vi "SendStartUpInitStatus.vi"(8 "error in (no error)":errorcluster, 10 "EDP Startup Init Status":T1, 11 "Handle In":u32 format="%x") -> (0 "error out":errorcluster, 3 "Handle Out":u32 format="%x")   [LabVIEW 2020]
uses:
  <userlib>/Beckhoff-LabVIEW-Interface/_DependsOn/With TypeResolving/Write Sync Single TypeResolved.vi
panel:
  in  "WriteGrpSymbols 2":string[](array[string])=["192.168.0.20.1.1:851::GVL_LabviewDataShare.in_bAardvarkBoardError_labview", "192.168.0.20.1.1:851::GVL_LabviewDataShare.in_bAsic1CalibrationCompleted_labview", "192.168.0.20.1.1:851::GVL_LabviewDataShare.in_bAsic1CalibrationInProgress_labview", "192.168.0.20.1.1:851::GVL_LabviewDataShare.in_bAsic1CalibrationSuccess_labview", "192.168.0.20.1.1:851::GVL_LabviewDataShare.in_bAsic1FFTCompleted_labview", "192.168.0.20.1.1:851::GVL_LabviewDataShare.in_bAsic1FFTInProgress_labview", "192.168.0.20.1.1:851::GVL_LabviewDataShare.in_bAsic1FFTSuccess_labview", "192.168.0.20.1.1:851::GVL_LabviewDataShare.in_bAsic2CalibrationCompleted_labview", "192.168.0.20.1.1:851::GVL_LabviewDataShare.in_bAsic2CalibrationInProgress_labview", "192.168.0.20.1.1:851::GVL_LabviewDataShare.in_bAsic2CalibrationSuccess_labview", "192.168.0.20.1.1:851::GVL_LabviewDataShare.in_bAsic2FFTCompleted_labview", "192.168.0.20.1.1:851::GVL_LabviewDataShare.in_bAsic2FFTInProgress_labview", "192.168.0.20.1.1:851::GVL_LabviewDataShare.in_bAsic2FFTSuccess_labview", "192.168.0.20.1.1:851::GVL_LabviewDataShare.in_bCalResultsDBStoreSuccess_labview", "192.168.0.20.1.1:851::GVL_LabviewDataShare.in_bFFTResultsDBStoreSuccess_labview", "192.168.0.20.1.1:851::GVL_LabviewDataShare.in_bLabviewHandshakeBit", "192.168.0.20.1.1:851::GVL_LabviewDataShare.in_bLabviewResetComplete_labview", "192.168.0.20.1.1:851::GVL_LabviewDataShare.in_bLabviewResetSuccess_labview", "192.168.0.20.1.1:851::GVL_LabviewDataShare.in_bNIDaqError_labview", "192.168.0.20.1.1:851::GVL_LabviewDataShare.in_bPTC04BoardError_labview", "192.168.0.20.1.1:851::GVL_LabviewDataShare.in_bStartupInitializationCompleted_labview", "192.168.0.20.1.1:851::GVL_LabviewDataShare.in_bStartupInitializationSuccess_labview", "192.168.0.20.1.1:851::GVL_LabviewDataShare.in_strAsic1SerialNo_labview", "192.168.0.20.1.1:851::GVL_LabviewDataShare.in_strAsic2SerialNo_labview"]
  out "Write Status 2":bool
  out "Has Matched? 2":bool
  out "Write Status":bool
  out "Has Matched?":bool
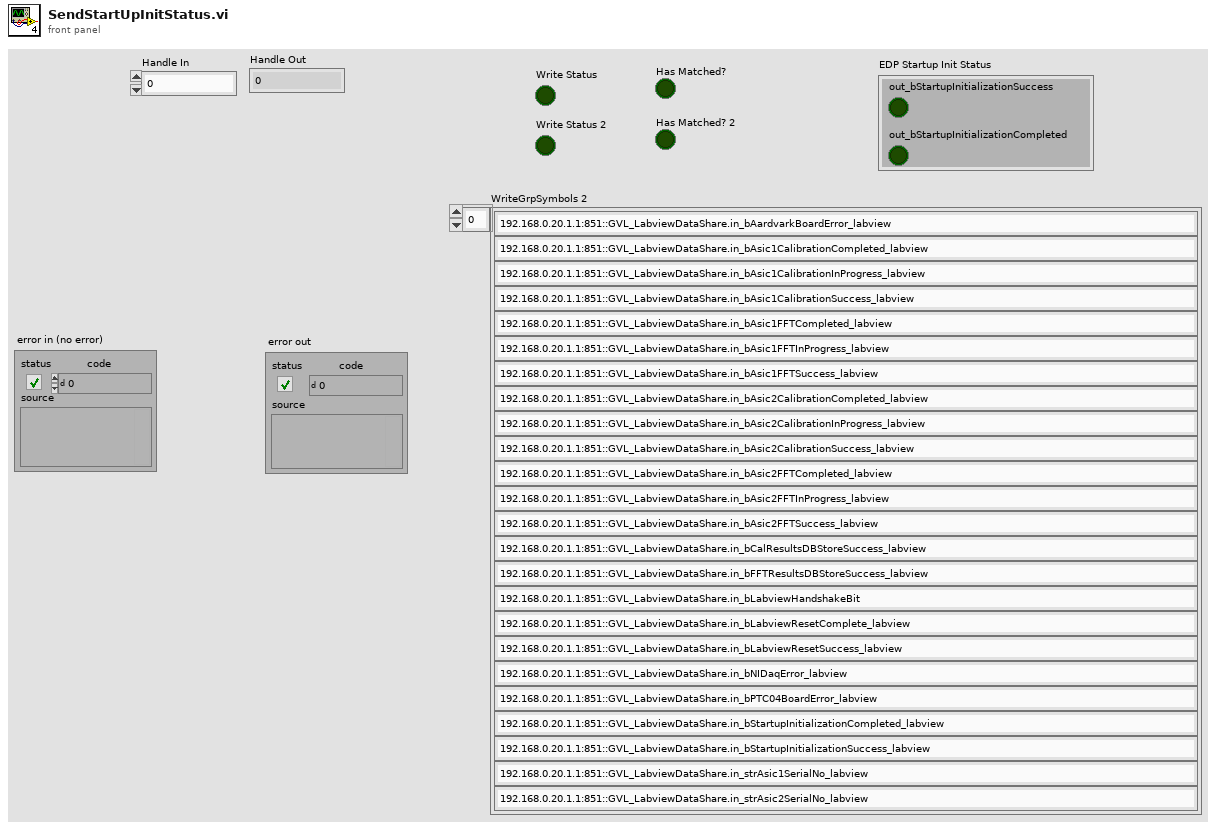
[diagram p1: front panel]
types:
  T1 = cluster{"out_bStartupInitializationSuccess":bool, "out_bStartupInitializationCompleted":bool}
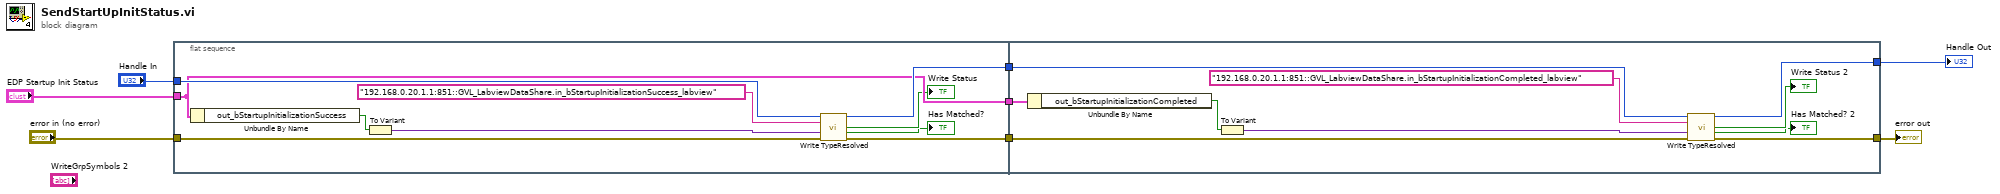
[diagram p0: block diagram]
diagram:
  n1 = flat-sequence {
    tunnel: "Handle In" -> [w18]
    tunnel: [w17] -> w8
    tunnel: [w16] -> w7
    tunnel: "error in (no error)" -> [w15]
    tunnel: "EDP Startup Init Status" -> [w12]
    tunnel: [w12] -> w6
    tunnel: w8 -> [w28]
    tunnel: w7 -> [w27]
    tunnel: w6 -> [w24]
    tunnel: [w20] -> w2
    tunnel: [w19] -> w1
    frame #0 {
      n2 = Unbundle By Name(w12) -> ("out_bStartupInitializationSuccess"=w14:bool)
      n3 = To Variant(anything=w14) -> (Variant=w13:variant)
      n4 = call-poly <userlib>:"Write TypeResolved.vi"("Handle"=w18, "SymbolName"="192.168.0.20.1.1:851::GVL_LabviewDataShare.in_bStartupInitializationSuccess_labview", "WData"=w13, "error constant"=w15) -> ("Handle"=w17:u32, "Write Status?"=→"Write Status":bool, "Has Matched?"=→"Has Matched?":bool, "error out"=w16:errorcluster)  [unwired: 8 in]
    }
    frame #1 {
      n5 = Unbundle By Name(w24) -> ("out_bStartupInitializationCompleted"=w26:bool)
      n6 = To Variant(anything=w26) -> (Variant=w25:variant)
      n7 = call-poly <userlib>:"Write TypeResolved.vi"("Handle"=w28, "SymbolName"="192.168.0.20.1.1:851::GVL_LabviewDataShare.in_bStartupInitializationCompleted_labview", "WData"=w25, "error constant"=w27) -> ("Handle"=w19:u32, "Write Status?"=→"Write Status 2":bool, "Has Matched?"=→"Has Matched? 2":bool, "error out"=w20:errorcluster)  [unwired: 8 in]
    }
  }
  "error out" <- w2
  "Handle Out" <- w1
